vi "Update ring names.vi"(8 "error in (no error)":errorcluster, 9 "Update from File-group-channel":bool, 10 "Names Array":string[](array[string]), 11 "MagLabGraph in":refnum<class "MagLabGraph.lvclass">) -> (0 "error out":errorcluster, 3 "MagLabGraph out":refnum<class "MagLabGraph.lvclass">)   [LabVIEW 2015, in "MagLabGraph.lvclass"]
uses:
  MagLabGraph.lvclass
  MagLabGraph.lvclass/MagLabGraph.ctl
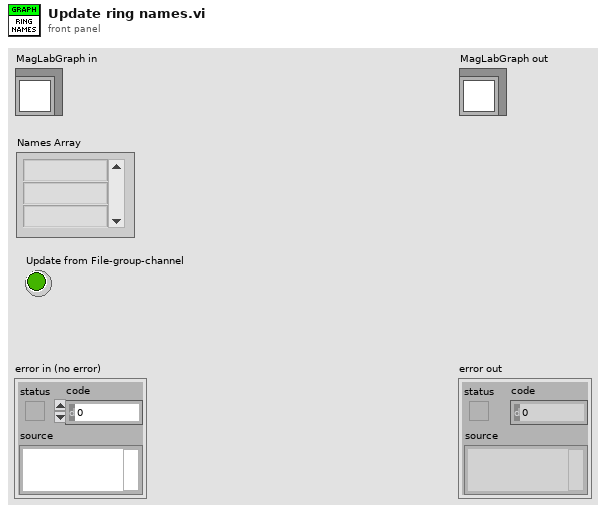
[diagram p1: front panel]
types:
  T1 = cluster{"File Path Control":path, "Group":string, "Channel":string, "Abbreviated":string}[]
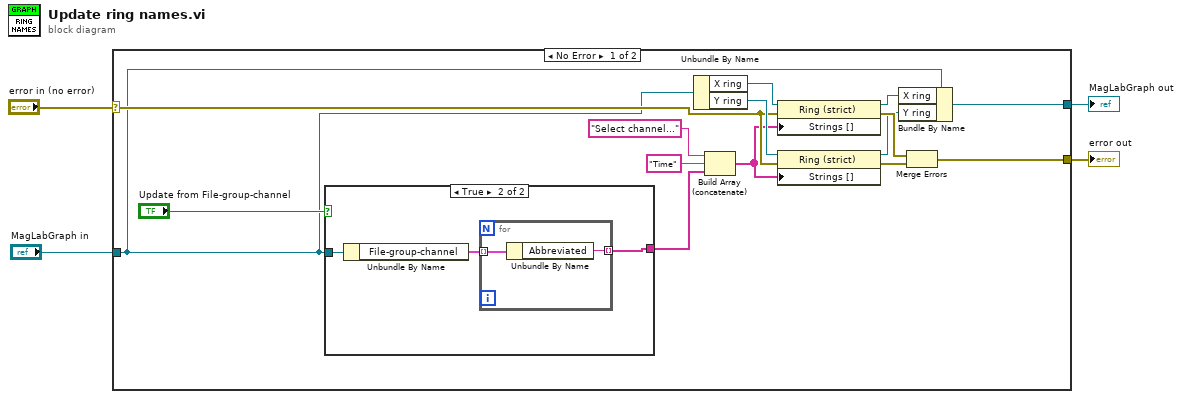
[diagram p0: block diagram]
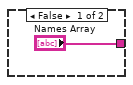
[diagram p2: hidden frame]
diagram:
  n1 = case shown="No Error" "error in (no error)" {
    selector: "error in (no error)" -> [w17 w27]
    tunnel: [w11 w27] -> w3
    tunnel: [w10 w26] -> w1
    tunnel: "MagLabGraph in" -> [w5 w26]
    frame No Error {
      n2 = case shown="True" "Update from File-group-channel" {
        tunnel: ["Names Array" w21] -> w16
        tunnel: w5 -> [_ w23]
        frame False {
        }
        frame True {
          n3 = Unbundle By Name(w23) -> ("File-group-channel"=w22:T1)
          n4 = for {
            tunnel: w22 -> [w25] mode=indexing
            tunnel: [w24] -> w21 mode=indexing
            n5 = Unbundle By Name(w25) -> ("Abbreviated"=w24:string)
          }
        }
      }
      n6 = Unbundle By Name(w5) -> ("X ring"=w19:refnum<vi>, "Y ring"=w18:refnum<vi>)
      n7 = Build Array (concatenate)("Select channel...", "Time" ("element"), w16) -> (w14:string[])
      n8 = property class="Ring (strict)"(reference=w19, error in=w17, "Strings []"=w14) -> (reference out=w9:refnum<vi>, error out=w13:errorcluster)
      n9 = property class="Ring (strict)"(reference=w18, error in=w17, "Strings []"=w14) -> (reference out=w8:refnum<vi>, error out=w12:errorcluster)
      n10 = Bundle By Name(cluster=w5, "X ring"=w9, "Y ring"=w8) -> (w10:refnum<class "MagLabGraph.lvclass">)
      n11 = Merge Errors(w13, w12) -> (w11:errorcluster)
    }
    frame Error {
    }
  }
  "error out" <- w3
  "MagLabGraph out" <- w1
